vi "HFRR ADV v024 new software.vi"() -> ()   [LabVIEW 2025] (continued)
            n3942 = Index Array(array=w5118, index #1=1 ("index")) -> (element #1=w5117:string, element #2=w5116:string, element #3=w5115:string, element #4=w5114:string, element #5=w5113:string, element #6=w5112:string)  [unwired: 5 in]
            n3943 = Index Array(array=w5108, index #1=1 ("index")) -> (element #1=w5107:string, element #2=w5106:string, element #3=w5105:string, element #4=w5104:string, element #5=w5103:string, element #6=w5102:string)  [unwired: 5 in]
            n3944 = Index Array(array=w5137, index #1=1 ("index")) -> (element #1=w5136:string, element #2=w5135:string, element #3=w5134:string, element #4=w5133:string, element #5=w5123:string, element #6=w5122:string)  [unwired: 5 in]
            n3945 = Index Array(array=w5057, index #1=1 ("index")) -> (element #1=w5089:string, element #2=w5088:string, element #3=w5087:string, element #4=w5086:string, element #5=w5085:string, element #6=w5084:string)  [unwired: 5 in]
            n3946 = local read "SEN.RUN HRS"() -> (w5060:dbl)
            n3947 = Divide(x=w5064, y=w5072) -> (x/y=w5071:dbl)
            n3948 = Increment(x=w5071) -> (x+1=w5067:dbl)
            n3949 = Number To Decimal String(number=w5067) -> (decimal integer string=→"run hrs":string)  [unwired: 1 in]
            n3950 = Divide(x=w5060, y=3600.0 ("f")) -> (x/y=w5055:dbl)
            n3951 = Round To Nearest(number=w5055) -> (nearest integer value=w5053:dbl)
            n3952 = Number To Decimal String(number=w5053) -> (decimal integer string=w5054:string)  [unwired: 1 in]
            n3953 = Number To Decimal String(number=w5062) -> (decimal integer string=w5063:string)  [unwired: 1 in]
            n3954 = local read "Model No"() -> (w5068:string)
            n3955 = local read "UUID"() -> (w5163:string)
            n3956 = local read "Serial No"() -> (w5167:string)
            n3957 = local read "Secret Key"() -> (w5168:string)
            n3958 = Concatenate Strings("\",\"MachineSerialNumber\":\"" ("string"), w5167) -> (w5171:string)
            n3959 = Concatenate Strings("\",\"ModelNumber\":\"" ("string"), w5068) -> (w5069:string)
            n3960 = Concatenate Strings("\",\"MachineRuntimeHours\":\"" ("string"), w5054) -> (w5172:string)
            n3961 = Concatenate Strings("\",\"MachineRuntimeCycles\":\"", w5063) -> (w5165:string)
            n3962 = Concatenate Strings(w5121, w5117) -> (w5151:string)
            n3963 = Concatenate Strings(w5120, w5107) -> (w5152:string)
            n3964 = Concatenate Strings(w5119, w5089) -> (w5150:string)
            n3965 = Concatenate Strings(w5171, w5069, w5172, w5165) -> (w5174:string)
            n3966 = Concatenate Strings(w5121, w5116) -> (w5148:string)
            n3967 = Concatenate Strings(w5120, w5106) -> (w5147:string)
            n3968 = Concatenate Strings(w5119, w5088) -> (w5149:string)
            n3969 = Concatenate Strings(w5121, w5115) -> (w5143:string)
            n3970 = Concatenate Strings(w5120, w5105) -> (w5144:string)
            n3971 = Concatenate Strings(w5119, w5087) -> (w5142:string)
            n3972 = Concatenate Strings(w5121, w5114) -> (w5140:string)
            n3973 = Concatenate Strings(w5120, w5104) -> (w5139:string)
            n3974 = Concatenate Strings(w5119, w5086) -> (w5141:string)
            n3975 = Concatenate Strings(w5151, w5152, w5150) -> (w5153:string)
            n3976 = Concatenate Strings(w5121, w5113) -> (w5130:string)
            n3977 = Concatenate Strings(w5120, w5103) -> (w5131:string)
            n3978 = Concatenate Strings(w5121, w5112) -> (w5127:string)
            n3979 = Concatenate Strings(w5120, w5102) -> (w5126:string)
            n3980 = Concatenate Strings(w5119, w5085) -> (w5129:string)
            n3981 = Concatenate Strings(w5119, w5084) -> (w5128:string)
            n3982 = Concatenate Strings("{\"SecretKey\":\"", w5168, w5174, "\",\"UUID\" : \"", w5163, "\",\"SensorInformation\":", "[{" ("string")) -> (w5101:string)
            n3983 = Concatenate Strings(w5148, w5147, w5149) -> (w5146:string)
            n3984 = Concatenate Strings(w5143, w5144, w5142) -> (w5145:string)
            n3985 = Concatenate Strings(w5140, w5139, w5141) -> (w5138:string)
            n3986 = Concatenate Strings(w5130, w5131, w5129) -> (w5132:string)
            n3987 = Concatenate Strings(w5127, w5126, w5128) -> (w5125:string)
            n3988 = Concatenate Strings(w5124, w5136, w5153, w5094) -> (w5100:string)
            n3989 = Concatenate Strings(w5124, w5135, w5146, w5094) -> (w5099:string)
            n3990 = Concatenate Strings(w5124, w5134, w5145, w5094) -> (w5098:string)
            n3991 = Concatenate Strings(w5124, w5133, w5138, w5094) -> (w5097:string)
            n3992 = Concatenate Strings(w5124, w5123, w5132, w5094) -> (w5096:string)
            n3993 = Concatenate Strings(w5124, w5122, w5125, "\"}" ("string")) -> (w5095:string)
            n3994 = Concatenate Strings(w5101, w5100, w5099, w5098, w5097, w5096, w5095, "]}" ("string")) -> (w5092:string)
            n3995 = local read "SEN.RUN HRS"() -> (w5059:dbl)
            n3996 = disable-structure shown="Disabled" {
              frame Disabled {
                n3997 = local read "state"() -> (w5178:string[])
                n3998 = Delete From Array(array=w5178, index=0) -> (array with subset deleted=w5176:string[])  [unwired: 1 in, 1 out]
                n3999 = for {
                  N: 6 -> [_]
                  tunnel: w5176 -> [w5189] mode=indexing
                  tunnel: [w5188] -> w5175 mode=indexing
                  n4000 = Equal?(x=w5189, y="Warning") -> (x = y?=w5185:bool)
                  n4001 = Equal?(x=w5189, y="Healthy") -> (x = y?=w5182:bool)
                  n4002 = Select(t="2" ("y"), s=w5185, f="3" ("y")) -> (s? t:f=w5180:string)
                  n4003 = Select(t="1" ("y"), s=w5182, f=w5180) -> (s? t:f=w5188:string)
                }
                "state1" <- w5175
              }
              frame Enabled {
              }
            }
            n4004 = stacked-sequence {
              tunnel: w5092 -> [w5200 _ _]
              tunnel: [_ _ w5216] -> _
              frame #0 {
                (unwired) FALSE ("convert eol (F)")
                w5202 = enum16{"start", "end", "current"}."start" ("pos mode (0:2)")
                n4005 = local read "Path"() -> (w5196:path)
                n4006 = Path To String(path=w5196) -> (string=w5208:string)
                n4007 = Concatenate Strings(w5208, "\\", "Sensor File Name") -> (w5209:string)
                n4008 = local write "standard output 2"(" ") -> ()
                n4009 = String To Path(string=w5209) -> (path=w5199:path)
                n4010 = call <vilib>:"Open_Create_Replace File.vi"("advisory dialog? (display:T)"=FALSE, "function (open:0)"=T32."create or replace", "file path"=w5199) -> ("error out"=w5212:errorcluster, "refnum"=w5211:refnum<file>)  [unwired: 5 in, 2 out]
                n4011 = Set File Position(refnum=w5211, from (0:start)=w5202, error in=w5212) -> (refnum out=w5192:refnum<file>, error out=w5191:errorcluster)  [unwired: 1 in]
                n4012 = Write to Binary File(file (use dialog)=w5192, data=" ", error in=w5191, 5:FALSE ("prepend array or string size? (T)")) -> (refnum out=w5203:refnum<file>, error out=w5204:errorcluster)  [unwired: 2 in, 1 out]
                n4013 = Set File Position(offset (in bytes) (0)=w5202, refnum=w5203, error in=w5204) -> (refnum out=w5195:refnum<file>, error out=w5194:errorcluster)  [unwired: 1 in]
                n4014 = Write to Binary File(file (use dialog)=w5195, data=w5200, error in=w5194, 5:FALSE ("prepend array or string size? (T)")) -> (error out=w5198:errorcluster)  [unwired: 2 in, 2 out]
                n4015 = flat-sequence {
                  tunnel: w5199 -> [w5214]
                  tunnel: w5198 -> [_]
                  frame #0 {
                    n4016 = call <vilib>:"Read Characters From File.vi"("file path (dialog if empty)"=w5214) -> ("character string"=→"Sensor Health JSON string":string)  [unwired: 5 in, 3 out]
                  }
                }
                "SinglePoint  2" <- w5200
              }
              frame #1 {
              }
              frame #2 {
                (unwired) "\"Stored\": true" ("string")
                n4017 = call <vilib>:"System Exec.vi"("run minimized? (F)"=TRUE, "wait until completion? (T)"=TRUE, "working directory"=path "C:/LAB-IQ-NXT", "command line"="C:\\LAB-IQ-NXT\\JPostH.bat") -> ("standard error"=→"Respose From Server 2":string, "standard output"=w5219:string)  [unwired: 4 in, 2 out]
                "standard output 2" <- w5219
                n4018 = Match Pattern(string=w5219, regular expression="JSONH Check String") -> (match substring=w5217:string, offset past match=w5216:i32)  [unwired: 1 in, 2 out]
                n4019 = Equal?(x=w5217, y="JSONH Check String") -> (x = y?=→"Upload \nConfirmed 2":bool)
              }
            }
            n4020 = Divide(x=w5059, y=3600.0 ("f")) -> (x/y=w5052:dbl)
            n4021 = local read "run time"() -> (w5109:string[])
            n4022 = Round To Nearest(number=w5052) -> (nearest integer value=w5051:dbl)
            n4023 = Number To Decimal String(number=w5051) -> (decimal integer string=w5050:string)  [unwired: 1 in]
            n4024 = Index Array(array="Sensor Information", index (col) #1=0 ("disabled index (col)"), index (col) #2=1 ("index (col)"), index (col) #3=2 ("index (col)"), index (col) #4=3 ("index (col)")) -> (element #1=→"Sensor name":string[], element #2=→"model num":string[], element #3=→"run time":string[], element #4=→"state":string[])  [unwired: 4 in]
            n4025 = Insert Into Array(array=w5109, index=1, new element #1=w5050, new element #2=w5050, new element #3=w5050, new element #4=w5050, new element #5=w5050, new element #6=w5050) -> (w5074:string[])
            "run" <- w5074
            n4026 = local read "out"() -> (w5056:string[])
            n4027 = local read "Sensor Information"() -> (w5076:string[][])
            n4028 = Replace Array Subset(array=w5076, new element #1=w5074, index (col) #1=2 ("disabled index (col)"), new element #2=w5056, index (col) #2=3 ("index (col)")) -> (w5075:string[][])  [unwired: 2 in]
            n4029 = local write "Sensor Information"(w5075) -> ()
          }
        }
        n4030 = case shown="True" w5023 {
          frame False {
          }
          frame True {
            n4031 = Equal?(x="FLAG", y=0.0) -> (x = y?=w5040:bool)
            n4032 = case shown="False" w5040 {
              frame False {
                n4033 = Get Date/Time In Seconds() -> (seconds since 1Jan1904=w5046:timestamp)
                n4034 = local read "START 2"() -> (w5044:dbl)
                n4035 = To Double Precision Float(number=w5046) -> (double precision float=w5045:dbl)
                n4036 = Subtract(x=w5045, y=w5044) -> (x-y=→"SENSOR TIME  2":dbl)
              }
              frame True {
                n4037 = Get Date/Time In Seconds() -> (seconds since 1Jan1904=w5048:timestamp)
                n4038 = To Double Precision Float(number=w5048) -> (double precision float=→"START 2":dbl)
                n4039 = local write "FLAG"(100.0 ("FLAG")) -> ()
              }
            }
          }
        }
        n4040 = disable-structure shown="Disabled" {
          disable-tunnel: w5026 -> [w5035 _]
          disable-tunnel: [w5034 _] -> w5025
          frame Disabled {
            n4041 = local read "Json St Flg"() -> (w5033:bool)
            n4042 = case shown="True" w5033 {
              tunnel: w5035 -> [w5036 w5038]
              tunnel: [w5036 w5037] -> w5034
              frame False {
              }
              frame True {
                n4043 = Increment(x=w5038) -> (x+1=w5037:dbl)
                "T cycle" <- w5037
                n4044 = local write "Json St Flg"(FALSE ("Json St Flg")) -> ()
              }
            }
          }
          frame Enabled {
          }
        }
        n4045 = local read "Quit"() -> (w5020:bool)
      }
    }
    frame Enabled {
    }
  }
  n4046 = stacked-sequence {
    tunnel: [w5418] -> w45
    frame #0 {
      w5418 = FALSE ("Upload \nConfirmed")
      n4047 = local write "Upload \nConfirmed"(w5418) -> ()
      n4048 = local write "St Str"("") -> ()
    }
  }
  n4049 = disable-structure shown="Disabled" {
    disable-tunnel: w45 -> [w5419 _]
    frame Disabled {
      n4050 = case shown="True" {
        selector: _ -> [_ _]
        tunnel: w5419 -> [_ w5420]
        frame False {
        }
        frame True {
          n4051 = while {
            tunnel: [w5426] -> _
            tunnel: w5420 -> [_]
            i -> [w5426]
            stop <- w5421 stop-if-true
            n4052 = local read "Json End Flg"() -> (w5425:bool)
            n4053 = Wait (ms)(milliseconds to wait=u32 20 ("Refresh Rate (ms)")) -> ()  [unwired: 1 out]
            n4054 = local read "refresh flag"() -> (w5422:bool)
            n4055 = local read "RUN"() -> (w5423:bool)
            n4056 = And(x=w5423, y=w5422) -> (x .and. y?=w5424:bool)
            n4057 = Or(x=w5424, y=w5425) -> (x .or. y?=w5427:bool)
            "AR Led" <- w5427
            n4058 = case shown="True" w5427 {
              frame False {
              }
              frame True {
                w5444 = "\",\""
                n4059 = local read "UUID"() -> (w5442:string)
                n4060 = local write "refresh flag"(FALSE ("refresh flag")) -> ()
                n4061 = local read "time"() -> (w5431:dbl)
                n4062 = Multiply(x=w5431, y=60.0) -> (x*y=w5430:dbl)
                n4063 = Concatenate Strings("UUID\" : \"", w5442, "\"}") -> (w5445:string)
                n4064 = Number To Fractional String(number=w5430, width (-)=i16 10, precision (6)=i16 4) -> (F-format string=w5459:string)  [unwired: 1 in]
                n4065 = Concatenate Strings("{", "\"Time\":\"", w5459, w5444) -> (w5454:string)
                n4066 = stacked-sequence {
                  tunnel: w5444 -> [w5507 w5515 w5522 w5530 w5538 w5547 w5554]
                  tunnel: [w5508 _ _ _ _ _ _] -> w5458
                  tunnel: [_ w5516 _ _ _ _ _] -> w5457
                  tunnel: [_ _ w5523 _ _ _ _] -> w5456
                  tunnel: [_ _ _ w5532 _ _ _] -> w5455
                  tunnel: w5445 -> [_ _ _ _ _ _ w5565]
                  tunnel: [_ _ _ _ _ _ w5564] -> w5441
                  tunnel: [_ _ _ _ _ w5544 _] -> w5440
                  tunnel: [_ _ _ _ w5537 _ _] -> w5439
                  frame #0 {
                    n4067 = local read "NORMAL LOAD"() -> (w5506:dbl)
                    n4068 = Number To Fractional String(number=w5506, width (-)=i16 10, precision (6)=i16 4) -> (F-format string=w5509:string)  [unwired: 1 in]
                    n4069 = Concatenate Strings("NormalLoad\":\"", w5509, w5507) -> (w5508:string)
                  }
                  frame #1 {
                    n4070 = local read "Temp"() -> (w5514:dbl)
                    n4071 = Number To Fractional String(number=w5514, width (-)=i16 10, precision (6)=i16 4) -> (F-format string=w5517:string)  [unwired: 1 in]
                    n4072 = Concatenate Strings("Temperature\":\"", w5517, w5515) -> (w5516:string)
                  }
                  frame #2 {
                    n4073 = local read "cof"() -> (w5520:dbl)
                    n4074 = Number To Fractional String(number=w5520, width (-)=i16 10, precision (6)=i16 4) -> (F-format string=w5524:string)  [unwired: 1 in]
                    n4075 = Concatenate Strings("FrictionalForce\":\"", w5524, w5522) -> (w5523:string)
                  }
                  frame #3 {
                    n4076 = local read "Set Hz"() -> (w5528:dbl)
                    n4077 = Multiply(x=w5528, y=60.0) -> (x*y=w5527:dbl)
                    n4078 = Number To Fractional String(number=w5527, width (-)=i16 10, precision (6)=i16 4) -> (F-format string=w5533:string)  [unwired: 1 in]
                    n4079 = Concatenate Strings("Speed\":\"", w5533, w5530) -> (w5532:string)
                  }
                  frame #4 {
                    n4080 = local read item#-1() -> (w5536)
                    n4081 = Number To Fractional String(number=w5536, width (-)=i16 10, precision (6)=i16 4) -> (F-format string=w5540:string)  [unwired: 1 in]
                    n4082 = Concatenate Strings("LinearDeformation\":\"", w5540, w5538) -> (w5537:string)
                  }
                  frame #5 {
                    n4083 = local read "AIR TEMP"() -> (w5543:dbl)
                    n4084 = local read "Json St Flg"() -> (w5545:bool)
                    n4085 = local read "Json End Flg"() -> (w5546:bool)
                    n4086 = Number To Fractional String(number=w5543, width (-)=i16 10, precision (6)=i16 4) -> (F-format string=w5549:string)  [unwired: 1 in]
                    n4087 = Concatenate Strings("Vibration\":\"", w5549, w5547) -> (w5544:string)
                    n4088 = And(x=w5545, y=w5546) -> ()  [unwired: 1 out]
                  }
                  frame #6 {
                    n4089 = local read "Json End Flg"() -> (w5553:bool)
                    n4090 = Get Date/Time In Seconds() -> (seconds since 1Jan1904=w5561:timestamp)
                    n4091 = local read "Json St Flg"() -> (w5552:bool)
                    n4092 = To Double Precision Float(number=w5561) -> (double precision float=w5560:dbl)
                    n4093 = Subtract(x=w5560, y=2082844800.0) -> (x-y=w5558:dbl)
                    n4094 = Number To Fractional String(number=w5558, width (-)=i16 12, precision (6)=i16 0) -> (F-format string=w5555:string)  [unwired: 1 in]
                    n4095 = case shown="True" w5553 {
                      tunnel: ["" w5568] -> w5562
                      tunnel: w5555 -> [_ w5569]
                      tunnel: w5554 -> [_ w5567]
                      frame False {
                      }
                      frame True {
                        n4096 = local write "Json End Flg"(FALSE ("Json St Flg")) -> ()
                        n4097 = Concatenate Strings("End\": \"", w5569, w5567) -> (w5568:string)
                      }
                    }
                    n4098 = case shown="True" w5552 {
                      tunnel: [w5572 w5575] -> w5563
                      tunnel: w5555 -> [_ w5576]
                      tunnel: w5554 -> [_ w5573]
                      frame False {
                        n4099 = local read "St Str"() -> (w5572:string)
                      }
                      frame True {
                        n4100 = Concatenate Strings("Start\":\"", w5576, w5573) -> (w5575:string)
                        "St Str" <- w5575
                        n4101 = local write "Json St Flg"(FALSE ("Json St Flg")) -> ()
                      }
                    }
                    n4102 = Concatenate Strings(w5563, w5562, w5565) -> (w5564:string)
                  }
                }
                n4103 = local read "FILE"() -> (w5433:string)
                n4104 = Concatenate Strings("\",\"OperatorID\":\"" ("string"), "Operator ID") -> (w5436:string)
                n4105 = Concatenate Strings("\",\"DatasetTitle\":\"" ("string"), w5433) -> (w5435:string)
                n4106 = Concatenate Strings("\",\"SerialNumber\":\"" ("string"), "Serial No") -> (w5465:string)
                n4107 = Concatenate Strings("\",\"ModelNumber\":\"" ("string"), "Model No") -> (w5464:string)
                n4108 = Concatenate Strings(w5465, w5464) -> (w5447:string)
                n4109 = Concatenate Strings("{\"SecretKey\":\"", "Secret Key", w5447, w5436, w5435, "\",\"Samples\":[") -> (w5452:string)
                n4110 = Concatenate Strings(w5454, w5458, w5457, w5456, w5455, w5439, w5440, w5441) -> (w5453:string)
                n4111 = Concatenate Strings(w5452, w5453, "]}") -> (w5451:string)
                n4112 = stacked-sequence {
                  tunnel: w5451 -> [w5480 _ _]
                  tunnel: [_ _ w5497] -> _
                  frame #0 {
                    (unwired) FALSE ("convert eol (F)")
                    w5482 = enum16{"start", "end", "current"}."start" ("pos mode (0:2)")
                    n4113 = Path To String(path="Path") -> (string=w5488:string)
                    n4114 = Concatenate Strings(w5488, "\\", "Data File Name") -> (w5490:string)
                    n4115 = local write "standard output"(" ") -> ()
                    n4116 = String To Path(string=w5490) -> (path=w5479:path)
                    n4117 = call <vilib>:"Open_Create_Replace File.vi"("advisory dialog? (display:T)"=FALSE, "function (open:0)"=T32."create or replace", "file path"=w5479) -> ("error out"=w5493:errorcluster, "refnum"=w5492:refnum<file>)  [unwired: 5 in, 2 out]
                    n4118 = Set File Position(refnum=w5492, from (0:start)=w5482, error in=w5493) -> (refnum out=w5473:refnum<file>, error out=w5472:errorcluster)  [unwired: 1 in]
                    n4119 = Write to Binary File(file (use dialog)=w5473, data=" ", error in=w5472, 5:FALSE ("prepend array or string size? (T)")) -> (refnum out=w5483:refnum<file>, error out=w5484:errorcluster)  [unwired: 2 in, 1 out]
                    n4120 = Set File Position(offset (in bytes) (0)=w5482, refnum=w5483, error in=w5484) -> (refnum out=w5476:refnum<file>, error out=w5475:errorcluster)  [unwired: 1 in]
                    n4121 = Write to Binary File(file (use dialog)=w5476, data=w5480, error in=w5475, 5:FALSE ("prepend array or string size? (T)")) -> (error out=w5478:errorcluster)  [unwired: 2 in, 2 out]
                    n4122 = flat-sequence {
                      tunnel: w5479 -> [w5495]
                      tunnel: w5478 -> [_]
                      frame #0 {
                        n4123 = call <vilib>:"Read Characters From File.vi"("file path (dialog if empty)"=w5495) -> ("character string"=→"JSON string":string)  [unwired: 5 in, 3 out]
                      }
                    }
                    "SinglePoint" <- w5480
                  }
                  frame #1 {
                  }
                  frame #2 {
                    (unwired) "\"Stored\": true" ("string")
                    n4124 = call <vilib>:"System Exec.vi"("run minimized? (F)"=TRUE, "wait until completion? (T)"=TRUE, "working directory"=path "C:/LAB-IQ-NXT", "command line"="C:\\LAB-IQ-NXT\\JPost.bat") -> ("standard error"=→"Respose From Server":string, "standard output"=w5500:string)  [unwired: 4 in, 2 out]
                    "standard output" <- w5500
                    n4125 = Match Pattern(string=w5500, regular expression="JSON Check String") -> (match substring=w5498:string, offset past match=w5497:i32)  [unwired: 1 in, 2 out]
                    n4126 = Equal?(x=w5498, y="JSON Check String") -> (x = y?=→"Upload \nConfirmed":bool)
                  }
                }
              }
            }
            n4127 = local read "Quit"() -> (w5421:bool)
          }
        }
      }
    }
    frame Enabled {
    }
  }
  n4128 = disable-structure shown="Disabled" {
    disable-tunnel: _ -> [w5583 _]
    frame Disabled {
      n4129 = while {
        shift-right: [w5591] -> w5579
        shift-left: _ -> [w5592]
        shift-right: [w5589] -> w5580
        shift-left: errorcluster {"status"=TRUE, "code"=0, "source"="Init"} ("error out") -> [w5590]
        shift-right: [w5587] -> _
        shift-left: "" -> [w5588]
        tunnel: [w5585] -> _
        tunnel: w5583 -> [_]
        i -> [w5585]
        stop <- w5584 stop-if-true
        n4130 = flat-sequence {
          tunnel: [w5593] -> w5586
          frame #0 {
            n4131 = Wait (ms)(milliseconds to wait=10.0 ("Delay")) -> (millisecond timer value=w5593:u32)
          }
        }
        n4132 = case shown="No Error" w5590 {
          selector: w5590 -> [w5623 w5742]
          tunnel: [w5606 w5744] -> w5591
          tunnel: [w5605 w5743] -> w5589
          tunnel: w5592 -> [w5624 w5736]
          tunnel: w5588 -> [w5604 w5735]
          tunnel: [w5603 w5735] -> w5587
          tunnel: w5586 -> [_ _]
          frame No Error {
            n4133 = Concatenate Strings("\r", "\n") -> (w5615:string)  [unwired: 1 in]
            n4134 = case shown="True" w5616 {
              tunnel: w5624 -> [w5648 w5655]
              tunnel: w5623 -> [w5647 w5654]
              tunnel: [w5648 w5653] -> w5622
              tunnel: [w5647 w5652] -> w5602
              tunnel: w5615 -> [_ w5651]
              frame False {
              }
              frame True {
                n4135 = VISA Write(VISA resource name=w5655, write buffer=w5651, error in (no error)=w5654) -> (VISA resource name out=w5653:refnum<visa-resource-name>, error out=w5652:errorcluster)  [unwired: 1 out]
                n4136 = local write "Read String"("") -> ()
                n4137 = local write item#-1(FALSE) -> ()
              }
            }
            n4138 = property class="Instr"(reference=w5622, error in=w5602) -> (reference out=w5621:refnum<visa-resource-name>, error out=w5620:errorcluster, "Serial Settings:Number of Bytes at Serial Port"=w5619:u32)
            n4139 = Greater?(x=w5619, y=u32 100) -> (0:w5617:bool)
            n4140 = case shown="True" w5617 {
              tunnel: w5621 -> [w5658 w5682]
              tunnel: w5620 -> [w5657 w5681]
              tunnel: w5619 -> [_ w5680]
              tunnel: [w5658 w5679] -> w5608
              tunnel: [w5657 w5678] -> w5607
              tunnel: w5604 -> [w5656 w5677]
              tunnel: [w5656 ""] -> w5603
              frame False {
              }
              frame True {
                w5667 = u32 6 ("y")
                # "Page 84 of \nmanual"
                n4141 = VISA Read(VISA resource name=w5682, byte count=w5680, error in (no error)=w5681) -> (VISA resource name out=w5679:refnum<visa-resource-name>, read buffer=w5675:string, error out=w5678:errorcluster)  [unwired: 1 out]
                n4142 = while {
                  tunnel: w5675 -> [w5731]
                  tunnel: [w5727] -> w5669 mode=indexing
                  tunnel: [w5721] -> w5673 mode=indexing
                  tunnel: [w5719] -> _
                  i -> [w5719]
                  stop <- w5724 stop-if-true
                  n4143 = String Subset(string=w5731, offset (0)=w5719) -> (substring=w5726:string)  [unwired: 1 in]
                  n4144 = String To Byte Array(string=w5726) -> (unsigned byte array=w5730:u8[])
                  n4145 = String Length(string=w5726) -> (length=w5725:i32)
                  n4146 = Index Array(array=w5730) -> (element=w5729:u8)  [unwired: 1 in]
                  n4147 = Equal To 0?(x=w5725) -> (x = 0?=w5724:bool)
                  n4148 = Number To Boolean Array(number=w5729) -> (Boolean array=w5723:bool[])
                  n4149 = Reverse 1D Array(array=w5723) -> (reversed array=w5722:bool[])
                  n4150 = And(x=w5723, y=bool[] [FALSE, FALSE, FALSE, FALSE, FALSE, FALSE, TRUE, TRUE] ("Boolean array")) -> (x .and. y?=w5727:bool[])
                  n4151 = And(x=w5722, y=bool[] [FALSE, FALSE, TRUE, TRUE, TRUE, TRUE, TRUE, TRUE] ("Boolean array")) -> (x .and. y?=w5721:bool[])
                }
                n4152 = Concatenate Strings(w5677, w5675) -> (→"Read String":string)
                n4153 = while {
                  tunnel: w5669 -> [w5718] mode=indexing
                  tunnel: [w5714] -> w5672
                  i -> [w5714]
                  stop <- w5715 stop-if-true
                  n4154 = Search 1D Array(1D array=w5718, element=TRUE) -> (index of element=w5716:i32)  [unwired: 1 in]
                  n4155 = Less Than 0?(x=w5716) -> (x < 0?=w5715:bool)
                }
                n4156 = Delete From Array(array=w5673, length=w5672, index (row)=0) -> (array with subset deleted=w5668:bool[][])  [unwired: 1 in, 1 out]
                n4157 = Array Size(array=w5668) -> (size(s)=w5670:i32[])
                n4158 = Index Array(array=w5670) -> (element=w5662:i32)  [unwired: 1 in]
                n4159 = Greater?(x=w5662, y=w5667) -> (0:w5665:bool)
                n4160 = Subtract(x=w5662, y=w5667) -> (x-y=w5666:u32)
                n4161 = Select(t=w5666, s=w5665, f=u32 0) -> (s? t:f=w5663:u32)
                n4162 = while {
                  tunnel: w5668 -> [w5701]
                  tunnel: [w5703] -> w5661 mode=indexing
                  tunnel: w5663 -> [w5685]
                  i -> [w5702]
                  stop <- w5700 stop-if-true
                  w5692 = 6 ("index")
                  w5691 = 2 ("length")
                  # "Page 65 of \nmanual"
                  n4163 = Multiply(x=u32 3 ("y"), y=w5702) -> (x*y=w5699:u32)
                  n4164 = Divide(x=u32 102 ("y"), y=u32 65520) -> (x/y=w5709:dbl)
                  n4165 = Greater Or Equal?(x=w5699, y=w5685) -> (x >= y?=w5700:bool)
                  n4166 = Index Array(array=w5701, index (row) #1=w5699) -> (element #1=w5697:bool[], element #2=w5696:bool[], element #3=w5695:bool[])  [unwired: 5 in]
                  n4167 = Reverse 1D Array(array=w5697) -> (reversed array=w5690:bool[])
                  n4168 = Reverse 1D Array(array=w5696) -> (reversed array=w5694:bool[])
                  n4169 = Reverse 1D Array(array=w5695) -> (reversed array=w5693:bool[])
                  n4170 = Delete From Array(array=w5690, length=w5691, index=w5692) -> (array with subset deleted=w5686:bool[])  [unwired: 1 out]
                  n4171 = Delete From Array(array=w5694, length=w5691, index=w5692) -> (array with subset deleted=w5687:bool[])  [unwired: 1 out]
                  n4172 = Delete From Array(array=w5693, length=w5691, index=w5692) -> (array with subset deleted=w5688:bool[])  [unwired: 1 out]
                  n4173 = Insert Into Array(array=bool[] [] ("Boolean array"), new element #1=w5686, new element #2=w5687, new element #3=w5688) -> (w5689:bool[])  [unwired: 1 in]
                  n4174 = Boolean Array To Number(Boolean array=w5689) -> (number=w5698:u32)
                  n4175 = Multiply(x=w5709, y=w5698) -> (x*y=w5708:dbl)
                  n4176 = Decrement(x=w5708) -> (x-1=w5707:dbl)
                  n4177 = Divide(x=w5707, y=u32 100) -> (x/y=w5705:dbl)
                  n4178 = Multiply(x=w5705, y=u32 10) -> (x*y=w5703:dbl)
                }
                n4179 = Delete From Array(array=w5661) -> (array with subset deleted=w5660:dbl[])  [unwired: 2 in, 1 out]
                "Waveform Graph 5" <- w5660
                "Waveform Chart 3" <- w5660
                n4180 = call-poly <vilib>:"Mean.vi"("X"=w5660) -> ("mean"=w5659:dbl)  [unwired: 1 out]
                n4181 = case shown="True" {
                  selector: _ -> [_ _]
                  tunnel: w5659 -> [_ w5684]
                  frame False {
                  }
                  frame True {
                    n4182 = local write item#-1(FALSE ("Zero 4")) -> ()
                    "z_measure" <- w5684
                  }
                }
              }
            }
            n4183 = local read item#-1() -> (w5599)
            n4184 = local read item#-1() -> (w5598)
            n4185 = local read item#-1() -> (w5600)
            n4186 = local read item#-1() -> (w5597)
            n4187 = case shown="True" w5595 {
              tunnel: w5599 -> [_ w5627]
              tunnel: w5600 -> [_ w5626]
              frame False {
              }
              frame True {
                n4188 = Build Array(w5627, w5626) -> (w5625:void[])
                n4189 = local read item#-1() -> (w5630)
                n4190 = Build Array (concatenate)(w5630, w5625) -> (w5628:void[])
                n4191 = local write item#-1(w5628) -> ()
                n4192 = local write item#-1(FALSE ("Boolean 8")) -> ()
              }
            }
            n4193 = call "Build XY Graph"("Enable"=w5597, "Reset"=w5598, "Y Input"=w5600, "X Input"=w5599) -> ("XY Graph"=w5596:cluster{"Y":dbl[], "Y":dbl[]}[])  [unwired: 6 in, 1 out]
            n4194 = case shown="True" {
              selector: _ -> [_ _]
              frame False {
              }
              frame True {
                n4195 = local read item#-1() -> (w5631)
                n4196 = Index Array(array=w5631, index (col) #1=0 ("disabled index (col)"), index (col) #2=1 ("index (col)")) -> (element #1=w5633, element #2=w5632)  [unwired: 2 in]
                n4197 = call <vilib>:"Linear Fit.vi"("Y"=w5633, "X"=w5632) -> ()  [unwired: 9 in, 5 out]
                n4198 = local write item#-1(FALSE ("Boolean 9")) -> ()
              }
            }
            n4199 = case shown="True" {
              selector: _ -> [_ _]
              frame False {
              }
              frame True {
                n4200 = local write item#-1(dbl[][] [] ("Captured Values")) -> ()
                n4201 = local write item#-1(FALSE ("Boolean 7")) -> ()
              }
            }
            n4202 = Concatenate Strings("\r", "\n") -> (w5610:string, w5609:string)
            n4203 = case shown="True" w5601 {
              tunnel: w5608 -> [w5640 w5646]
              tunnel: w5607 -> [w5639 w5645]
              tunnel: [w5640 w5644] -> w5606
              tunnel: [w5639 w5643] -> w5605
              tunnel: w5610 -> [_ w5642]
              frame False {
              }
              frame True {
                n4204 = VISA Write(VISA resource name=w5646, write buffer=w5642, error in (no error)=w5645) -> (VISA resource name out=w5644:refnum<visa-resource-name>, error out=w5643:errorcluster)  [unwired: 1 out]
                n4205 = local write item#-1(FALSE ("WRITE")) -> ()
              }
            }
          }
          frame Error {
            w5734 = u16 10 items=["1.0"=10, "1.5"=15, "2.0"=20] ("stop bits (10: 1 bit)")
            n4206 = Wait (ms)(milliseconds to wait=u32 20) -> ()  [unwired: 1 out]
            n4207 = VISA Close(VISA resource name=w5736, error in (no error)=w5742) -> (error out=w5741:errorcluster)
            n4208 = call <vilib>:"Clear Errors.vi"("error in (no error)"=w5741) -> ("error out"=w5740:errorcluster)  [unwired: 5 in, 1 out]
            n4209 = call-poly "VISA Configure Serial Port"("timeout (10sec)"=u32 200, "Enable Termination\nChar (T)"=TRUE ("Enable Termination\nChar (T)"), "baud rate (9600)"=u32 921600, "error in (no error)"=w5740, "stop bits (10: 1 bit)"=w5734) -> ("VISA resource name"=w5732:refnum<visa-resource-name>, "VISA resource name out"=w5744:refnum<visa-resource-name>, "error out"=w5743:errorcluster)  [unwired: 8 in]
          }
        }
        n4210 = local read "Quit"() -> (w5584:bool)
      }
      n4211 = VISA Close(VISA resource name=w5579, error in (no error)=w5580) -> (error out=w5578:errorcluster)
      n4212 = call <vilib>:"Clear Errors.vi"("error in (no error)"=w5578) -> ()  [unwired: 5 in, 2 out]
    }
    frame Enabled {
    }
  }
  n4213 = disable-structure shown="Disabled" {
    disable-tunnel: _ -> [w5749 _]
    frame Disabled {
      n4214 = while {
        tunnel: [w5756] -> _
        shift-right: [w5753] -> w5746
        shift-left: _ -> [w5755]
        shift-right: [w5754] -> w5747
        shift-left: errorcluster {"status"=TRUE, "code"=0, "source"="Init"} ("error out") -> [w5752]
        tunnel: w5749 -> [_]
        i -> [w5756]
        stop <- w5750 stop-if-true
        n4215 = flat-sequence {
          tunnel: w5752 -> [w5847]
          tunnel: [w5847] -> w5751
          frame #0 {
            n4216 = Wait (ms)(milliseconds to wait=u32 50) -> ()  [unwired: 1 out]
          }
        }
        n4217 = case shown="No Error" w5751 {
          selector: w5751 -> [w5797 w5840]
          tunnel: w5755 -> [w5796 w5839]
          tunnel: [w5763 w5830] -> w5754
          tunnel: [w5764 w5838] -> w5753
          frame No Error {
            w5790 = T33 {"Mode"=enum."RTU", "Slave Address"=1} ("Serial Parameters")
            n4218 = call-poly <vilib>:"MB Serial Master Query (poly).vi"("VISA resource name"=w5796, "Starting Address"=i16 1000, "Quantity"=u16 1, "Timeout"=u32 1000, "error in"=w5797, "Serial Parameters"=w5790) -> ("VISA resource name out"=w5791:refnum<visa-resource-name>, "Input Registers"=w5793:u16[], "error out"=w5789:errorcluster)  [unwired: 10 in, 1 out]
            n4219 = Random Number (0-1)() -> (number: 0 to 1=w5778:dbl)
            n4220 = Index Array(array=w5793, index=0) -> (element=w5788:u16)
            n4221 = Subtract(x=w5778, y=0.5) -> (x-y=w5777:dbl)
            n4222 = Divide(x=w5788, y=10 ("index")) -> (x/y=w5782:dbl)
            n4223 = Multiply(x=w5777, y=0.5) -> (x*y=w5776:dbl)
            n4224 = Add(x=w5782, y=w5776) -> (x+y=w5781:dbl)
            n4225 = local read "Amb temp"() -> (w5765:dbl)
            n4226 = Multiply(x=w5781, y=0.2) -> (x*y=w5785:dbl)
            n4227 = Multiply(x=w5765, y=0.8) -> (x*y=w5783:dbl)
            n4228 = Add(x=w5785, y=w5783) -> (x+y=w5766:dbl)
            n4229 = local read "set temp old"() -> (w5760:dbl)
            n4230 = local write "Amb temp"(w5766) -> ()
            n4231 = Select(t="SetTemp 2", s="Heater", f=100.0) -> (s? t:f=w5761:dbl)
            n4232 = Not Equal?(x=w5761, y=w5760) -> (x != y?=w5759:bool)
            n4233 = case shown="True" w5759 {
              tunnel: w5791 -> [w5825 w5827]
              tunnel: [w5824 w5827] -> w5771
              tunnel: w5789 -> [w5823 w5826]
              tunnel: [w5822 w5826] -> w5769
              tunnel: w5761 -> [w5817 _]
              tunnel: w5790 -> [w5819 w5828]
              tunnel: [w5819 w5828] -> w5772
              frame True {
                n4234 = Multiply(x=w5817, y=10 ("index")) -> (x*y=w5816:dbl)
                n4235 = call-poly <vilib>:"MB Serial Master Query (poly).vi"("VISA resource name"=w5825, "Address"=u16 0, "Holding Register"=w5816, "Timeout"=u32 1000, "error in"=w5823, "Serial Parameters"=w5819) -> ("VISA resource name out"=w5824:refnum<visa-resource-name>, "error out"=w5822:errorcluster)  [unwired: 11 in, 1 out]
                "set temp old" <- w5817
              }
              frame False {
              }
            }
            n4236 = flat-sequence {
              tunnel: [w5798] -> _
              tunnel: [w5798] -> w5768
              tunnel: w5769 -> [w5798]
              frame #0 {
                n4237 = Wait (ms)(milliseconds to wait=u32 100) -> ()  [unwired: 1 out]
              }
            }
            n4238 = call "Elapsed Time12"("Time Target (s)"=2.0, "Auto Reset"=TRUE) -> ("Time has Elapsed"=w5773:bool)  [unwired: 10 in, 7 out]
            n4239 = case shown="True" w5773 {
              tunnel: w5772 -> [w5802 w5815]
              tunnel: [w5802 w5815] -> _
              tunnel: [w5801 w5813] -> w5764
              tunnel: w5771 -> [w5801 w5814]
              tunnel: [w5800 w5811] -> w5763
              tunnel: w5768 -> [w5800 w5812]
              frame False {
              }
              frame True {
                n4240 = call-poly <vilib>:"MB Serial Master Query (poly).vi"("VISA resource name"=w5814, "Starting Address"=i16 1003 ("Addr"), "Quantity"=u16 1, "Timeout"=u32 1000, "error in"=w5812, "Serial Parameters"=w5815) -> ("VISA resource name out"=w5813:refnum<visa-resource-name>, "Input Registers"=w5808:u16[], "error out"=w5811:errorcluster)  [unwired: 10 in, 1 out]
                n4241 = Index Array(array=w5808, index=0) -> (element=w5807:u16)
                n4242 = Divide(x=w5807, y=u16 10) -> (x/y=w5803:dbl)
                n4243 = local write "set temp old"(w5803) -> ()
                n4244 = local write "SetTemp"(w5803) -> ()
              }
            }
            "Error Code" <- w5763
            n4245 = Unbundle(w5763) -> ("status"=→"TK4 status":bool)  [unwired: 2 out]
            "SetTemp" <- "SetTemp 2"
          }
          frame Error {
            w5842 = u16 0 items=["None", "Odd", "Even", "Mark", "Space"] ("Parity")
            w5843 = u16 0 items=["None", "XON/XOFF", "RTS/CTS", "XON/XOFF & RTS/CTS", "DTR/DSR", "XON/XOFF & DTR/DSR"] ("Flow Control")
            n4246 = VISA Clear(VISA resource name=w5839, error in (no error)=w5840) -> (VISA resource name out=w5833:refnum<visa-resource-name>, error out=w5831:errorcluster)
            n4247 = VISA Close(VISA resource name=w5833, error in (no error)=w5831) -> (error out=w5832:errorcluster)
            n4248 = call <vilib>:"Clear Errors.vi"("error in (no error)"=w5832) -> ("error out"=w5841:errorcluster)  [unwired: 5 in, 1 out]
            n4249 = Unbundle By Name(T33 {"Mode"=enum."RTU", "Slave Address"=1} ("input cluster")) -> ("Mode"=w5844:enum16{"RTU", "ASCII"})
            n4250 = call <vilib>:"MB Serial Init.vi"("Timeout"=u32 100, "Flow Control"=w5843, "Mode"=w5844, "error in (no error)"=w5841, "Parity"=w5842, "Baud Rate"=u32 9600, "VISA resource name"="Lubrication System COM Port :") -> ("error out"=w5830:errorcluster, "VISA resource name out"=w5838:refnum<visa-resource-name>)  [unwired: 3 in]
            n4251 = local write "set temp old"(0.0 ("set temp old")) -> ()
            n4252 = Unbundle(w5830) -> ("status"=w5829:bool)  [unwired: 2 out]
            n4253 = case shown="True" w5829 {
              selector: w5829 -> [_ w5846]
              frame False {
              }
              frame True {
                n4254 = local write "TK4 status"(w5846) -> ()
              }
            }
          }
        }
        n4255 = local read "Quit"() -> (w5750:bool)
      }
      n4256 = VISA Close(VISA resource name=w5746, error in (no error)=w5747) -> (error out=w5745:errorcluster)
      n4257 = call <vilib>:"Clear Errors.vi"("error in (no error)"=w5745) -> ()  [unwired: 5 in, 2 out]
    }
    frame Enabled {
    }
  }
